vi "VALIDATE_VENDING MACHINE.vi"(7 "TYPE ?":bool, 8 "error in (no error)":errorcluster, 10 "PRODUCTS":T1, 11 "MONEY":T2) -> (0 "error out":errorcluster, 1 "Valido?":bool, 2 "PRODUCTS OUT":T1, 3 "MONEY OUT":T2)   [LabVIEW 2019, in "DB_VENDING MACHINE.lvlib"]
doc: "Aquí realizamos la validación de los ususarios"
uses:
  DB_VENDING MACHINE.lvlib
  Type Defs/MONEY.ctl
  Type Defs/PRODUCTS.ctl
  <vilib>/addons/database/_DB Variant To Data/Database Variant To Data.xnode
  <vilib>/addons/database/NI_Database_API.lvlib
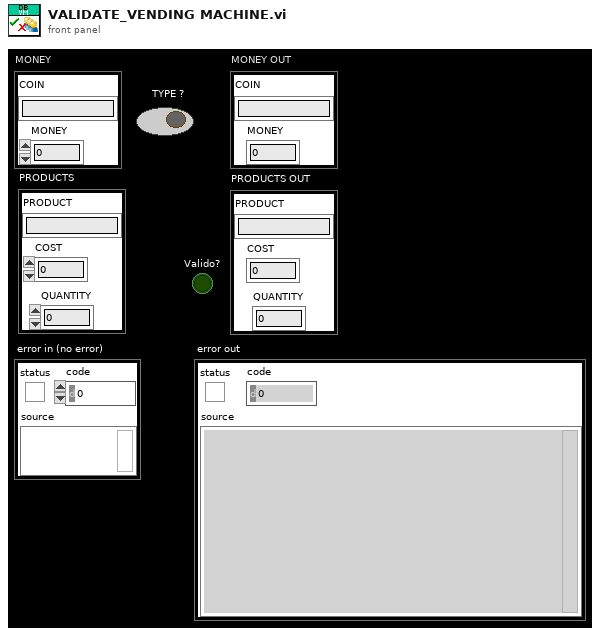
[diagram p1: front panel]
types:
  T1 = typedef "DB_VENDING MACHINE.lvlib/PRODUCTS.ctl" = cluster{"PRODUCT":string, "COST":dbl, "QUANTITY":i8}
  T2 = typedef "DB_VENDING MACHINE.lvlib/MONEY.ctl" = cluster{"COIN":string, "MONEY":dbl}
  T3 = typedef "NI_Database_API.lvlib/Conn ObjectReference.ctl" = refnum<k1>
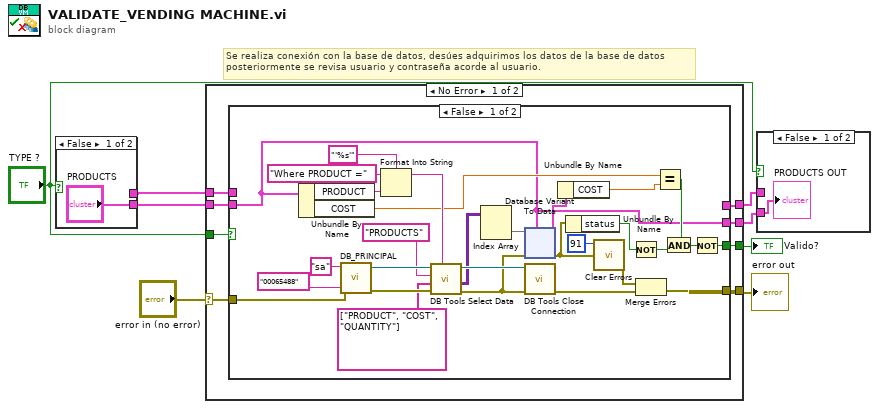
[diagram p0: block diagram]
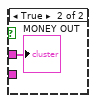
[diagram p2: hidden frame]
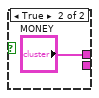
[diagram p3: hidden frame]
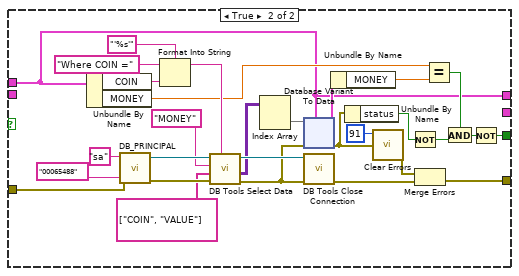
[diagram p4: hidden frame]
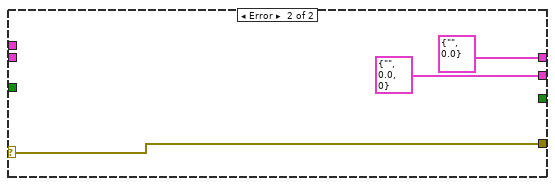
[diagram p5: hidden frame]
diagram:
  # "Se realiza conexión con la base de datos, desúes adquirimos los datos de la base de datos\nposteriormente se revisa usuario y contraseña acorde al usuario."
  n1 = case shown="False" "TYPE ?" {
    tunnel: ["PRODUCTS" _] -> w4
    tunnel: [_ "MONEY"] -> w5
    frame False {
    }
    frame True {
    }
  }
  n2 = case shown="No Error" "error in (no error)" {
    selector: "error in (no error)" -> [w18 w242]
    tunnel: w5 -> [w17 _]
    tunnel: [w16 w242] -> w8
    tunnel: [w12 T2 {"COIN"="", "MONEY"=0.0} ("MONEY")] -> w2
    tunnel: [w15 _] -> w6
    tunnel: w4 -> [w14 _]
    tunnel: [w13 T1 {"PRODUCT"="", "COST"=0.0, "QUANTITY"=0} ("PRODUCTS")] -> w1
    tunnel: "TYPE ?" -> [w11 _]
    frame No Error {
      n3 = case shown="False" w11 {
        tunnel: w18 -> [w25 w165]
        tunnel: w17 -> [_ w146]
        tunnel: [w24 w154] -> w16
        tunnel: [w20 w145] -> w15
        tunnel: [_ w146] -> w12
        tunnel: w14 -> [w19 _]
        tunnel: [w19 _] -> w13
        frame False {
          n4 = Unbundle By Name(w19) -> ("PRODUCT"=w38:string, "COST"=w28:dbl)
          n5 = call "DB_PRINCIPAL.vi"("error in (no error)"=w25, "password"="00065488", "userID"="sa") -> ("error out"=w46:errorcluster, "connection reference"=w47:T3)  [unwired: 7 in]
          n6 = Format Into String(format string="'%s'", initial string="Where PRODUCT =" ("condition"), w38) -> (resulting string=w36:string)  [unwired: 1 in, 1 out]
          n7 = call <vilib>:"DB Tools Select Data.vi"("condition"=w36, "error in (no error)"=w46, "columns"=string[] ["PRODUCT", "COST", "QUANTITY"], "table"="PRODUCTS", "connection reference"=w47) -> ("error out"=w33:errorcluster, "data"=w35:variant[][], "connection reference out"=w45:T3)  [unwired: 1 in]
          n8 = Index Array(array=w35) -> (element=w34:variant[])  [unwired: 2 in]
          n9 = xnode "Database Variant To Data"("database variant"=w34, "error in (no error)"=w33, "type"=w19) -> ("data"=w21:T1, "error out"=w31:errorcluster)
          n10 = call <vilib>:"DB Tools Close Connection.vi"("error in (no error)"=w33, "connection reference"=w45) -> ("error out"=w40:errorcluster)  [unwired: 5 in]
          n11 = Unbundle By Name(w21) -> ("COST"=w23:dbl)
          n12 = Unbundle By Name(w31) -> ("status"=w32:bool)
          n13 = call <vilib>:"Clear Errors.vi"("error in (no error)"=w31, "specific error code to clear (0: all)"=91) -> ("error out"=w29:errorcluster)  [unwired: 4 in, 1 out]
          n14 = Not(x=w32) -> (.not. x?=w27:bool)
          n15 = Merge Errors(w29, w40) -> (w24:errorcluster)
          n16 = Equal?(x=w28, y=w23) -> (x = y?=w26:bool)
          n17 = And(x=w26, y=w27) -> (x .and. y?=w22:bool)
          n18 = Not(x=w22) -> (.not. x?=w20:bool)
        }
        frame True {
          n19 = Unbundle By Name(w146) -> ("COIN"=w163:string, "MONEY"=w152:dbl)
          n20 = call "DB_PRINCIPAL.vi"("error in (no error)"=w165, "password"="00065488", "userID"="sa") -> ("error out"=w172:errorcluster, "connection reference"=w173:T3)  [unwired: 7 in]
          n21 = Format Into String(format string="'%s'", initial string="Where COIN =" ("condition"), w163) -> (resulting string=w161:string)  [unwired: 1 in, 1 out]
          n22 = call <vilib>:"DB Tools Select Data.vi"("condition"=w161, "error in (no error)"=w172, "columns"=string[] ["COIN", "VALUE"], "table"="MONEY", "connection reference"=w173) -> ("error out"=w158:errorcluster, "data"=w160:variant[][], "connection reference out"=w171:T3)  [unwired: 1 in]
          n23 = Index Array(array=w160) -> (element=w159:variant[])  [unwired: 2 in]
          n24 = xnode "Database Variant To Data"("database variant"=w159, "error in (no error)"=w158, "type"=w146) -> ("data"=w148:T2, "error out"=w156:errorcluster)
          n25 = call <vilib>:"DB Tools Close Connection.vi"("error in (no error)"=w158, "connection reference"=w171) -> ("error out"=w166:errorcluster)  [unwired: 5 in]
          n26 = Unbundle By Name(w148) -> ("MONEY"=w147:dbl)
          n27 = Unbundle By Name(w156) -> ("status"=w157:bool)
          n28 = call <vilib>:"Clear Errors.vi"("error in (no error)"=w156, "specific error code to clear (0: all)"=91) -> ("error out"=w153:errorcluster)  [unwired: 4 in, 1 out]
          n29 = Not(x=w157) -> (.not. x?=w150:bool)
          n30 = Merge Errors(w153, w166) -> (w154:errorcluster)
          n31 = Equal?(x=w152, y=w147) -> (x = y?=w149:bool)
          n32 = And(x=w149, y=w150) -> (x .and. y?=w151:bool)
          n33 = Not(x=w151) -> (.not. x?=w145:bool)
        }
      }
    }
    frame Error {
    }
  }
  "error out" <- w8
  "Valido?" <- w6
  n34 = case shown="False" "TYPE ?" {
    tunnel: w2 -> [_ w244]
    tunnel: w1 -> [w243 _]
    frame False {
      "PRODUCTS OUT" <- w243
    }
    frame True {
      "MONEY OUT" <- w244
    }
  }
